vi "send get to epics.vi"(6 "to PROC?":bool, 7 "Command":string="status", 8 "error in":errorcluster, 10 "Param Cluster":T3={"Card"=1, "Num Dev"=1}, 11 "IOC":string) -> (0 "error out":errorcluster, 1 "Status":bool, 3 "Data Value Out":T2, 4 "PV Info":T1[](array[typedef]))   [LabVIEW 2022 SP3]
uses:
  pectus/control/Param Epics Cluster.ctl
  pectus/control/epics value.ctl
  Program Files/National Instruments/LabVIEW 2023/user.lib/calab/PV Info.ctl
  Program Files/National Instruments/LabVIEW 2023/user.lib/calab/CaLab.lvlib
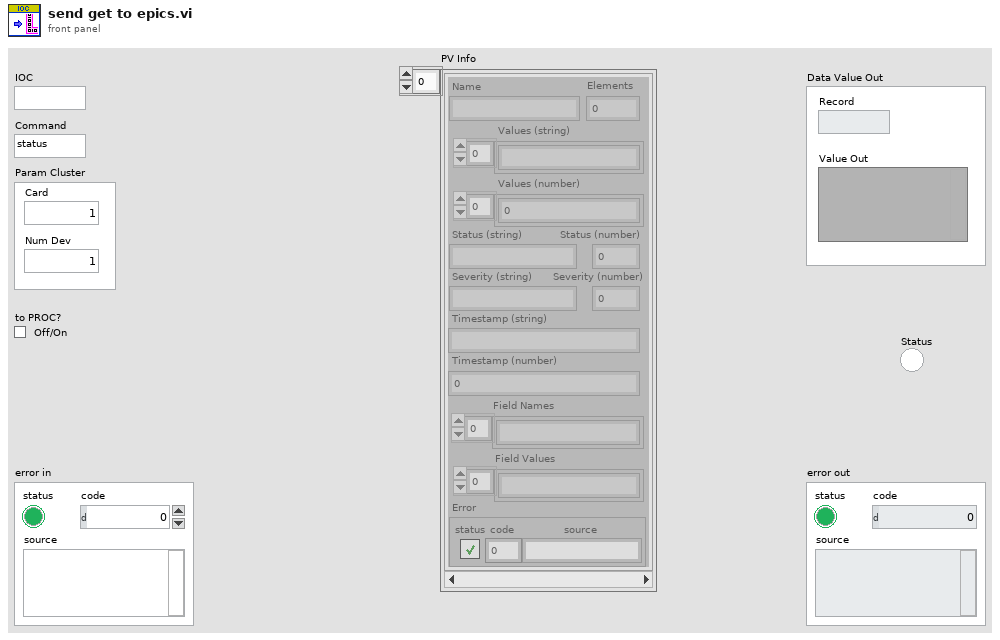
[diagram p1: front panel]
types:
  T1 = typedef "CaLab.lvlib/PV Info.ctl" = cluster{"Name":string, "Elements":i32, "Values (string)":string[], "Values (number)":dbl[], "Status (string)":string, "Status (number)":i16, "Severity (string)":string, "Severity (number)":i16, "Timestamp (string)":string, "Timestamp (number)":i32, "Field Names":string[], "Field Values":string[], "Error":errorcluster}
  T2 = typedef "epics value.ctl" = cluster{"Record":string, "Value Out":variant}
  T3 = typedef "Param Epics Cluster.ctl" = cluster{"Card":u16, "Num Dev":u16}
  T4 = typedef "ca cluster.ctl" = cluster{"record":string, "prefix":string, "CA":string}
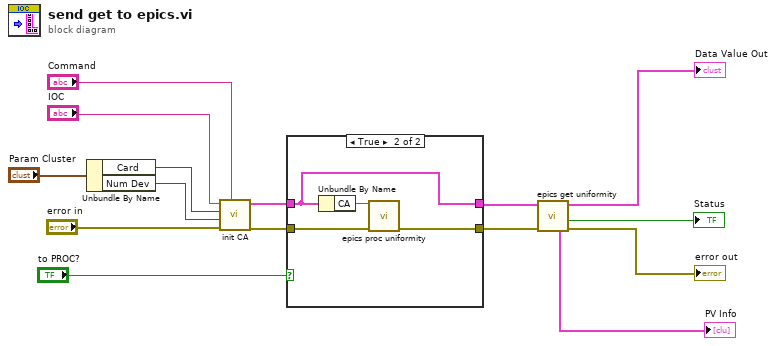
[diagram p0: block diagram]
diagram:
  n1 = Unbundle By Name("Param Cluster") -> ("Card"=w11:u16, "Num Dev"=w10:u16)
  n2 = call "init CA.vi"("Command"="Command", "error in"="error in", "Device"=w10, "Card"=w11, "IOC"="IOC") -> ("error out"=w9:errorcluster, "CA out"=w8:T4)  [unwired: 5 in]
  n3 = case shown="True" "to PROC?" {
    tunnel: w9 -> [w16 w21]
    tunnel: w8 -> [w17 w19]
    tunnel: [w17 w19] -> w5
    tunnel: [w16 w18] -> w6
    frame False {
    }
    frame True {
      n4 = Unbundle By Name(w19) -> ("CA"=w20:string)
      n5 = call "epics proc uniformity.vi"("error in"=w21, "CA to PROC"=w20) -> ("error out"=w18:errorcluster)  [unwired: 9 in]
    }
  }
  n6 = call "epics get uniformity.vi"("error in"=w6, "CA in"=w5) -> ("error out"=→"error out":errorcluster, "Status"=→"Status":bool, "Data Value Out"=→"Data Value Out":T2, "PV Info"=→"PV Info":T1[])  [unwired: 5 in, 1 out]
